vi "IMAQ FPGA Camera Link 8 Tap 10-Bit.vi"(6 "Ready for Output":bool=TRUE, 7 "Camera Link Enables":T3, 8 "Cancel Acquisition":bool, 9 "Acquire":bool=TRUE, 10 "Camera Link Data":T2, 11 "Acquisition Settings":T4) -> (0 "Output Valid":bool, 2 "Acquisition Status":T1, 3 "Vision Pixel Bus Out":T5={"Pixel Data"=[0, 0, 0, 0, 0, 0, 0, 0], "DV"=[FALSE, FALSE, FALSE, FALSE, FALSE, FALSE, FALSE, FALSE], "EOL"=FALSE, "EOI"=FALSE, "Data Type"=enum."U16 x 8"}, 5 "Acquisition Overflow":bool)   [LabVIEW 2017]
doc: "Acquires images from an 8 tap 10-bit (1X8-1Y) Camera Link Camera. On each pixel clock, 8 adjacent pixels arrive starting at the left of the image. Ensure that this VI is called from a Single Cycle Timed Loop that is running faster than the pixel clock of the camera.\n\nThe <B>Vision Pixel Bus Out</B> can be connected to Vision FPGA algorithms for processing."
uses:
  <vilib>/visionFPGA/Controls/IMAQ FPGA Pixel Bus u16x8.ctl
  <vilib>/visionFPGA/Basics/Camera Link Acquisition/Pixel Bus to Vision Pixel Bus/IMAQ FPGA Camera Link Pixel Bus to Vision Pixel Bus U16x8.vi
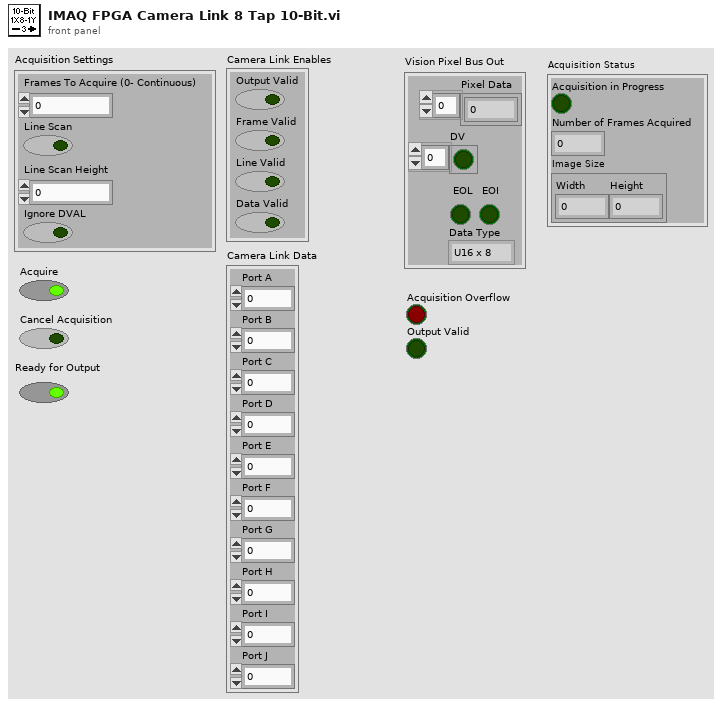
[diagram p1: front panel]
types:
  T1 = cluster{"Acquisition in Progress":bool, "Number of Frames Acquired":u32, "Image Size":cluster{"Width":u32, "Height":u32}}
  T2 = cluster{"Port A":u8, "Port B":u8, "Port C":u8, "Port D":u8, "Port E":u8, "Port F":u8, "Port G":u8, "Port H":u8, "Port I":u8, "Port J":u8}
  T3 = cluster{"Output Valid":bool, "Frame Valid":bool, "Line Valid":bool, "Data Valid":bool}
  T4 = cluster{"Frames To Acquire (0- Continuous)":u32, "Line Scan":bool, "Line Scan Height":u32, "Ignore DVAL":bool}
  T5 = typedef "IMAQ FPGA Pixel Bus u16x8.ctl" = cluster{"Pixel Data":u16[], "DV":bool[], "EOL":bool, "EOI":bool, "Data Type":enum16{"U16 x 8"}}
  T6 = cluster{"Acquisition in Progress":bool, "Num Frames Acquired":u32, "Height":u32, "Number of Cycles per Line":u32}
  T7 = cluster{"Acquisition in Progress":bool, "Num Frames Acquired":u32, cluster{u32, "Height":u32}}
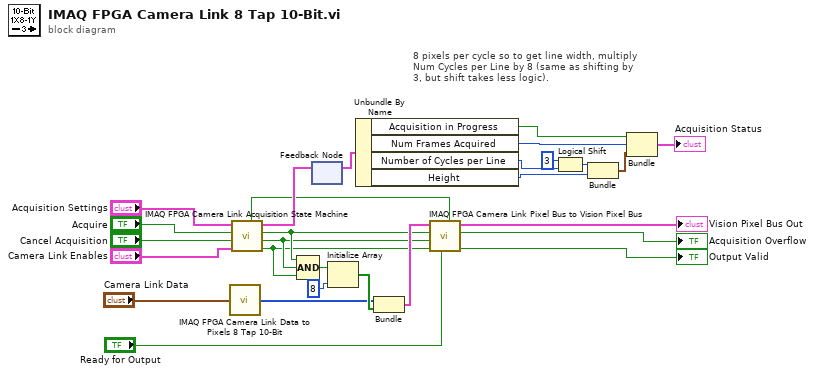
[diagram p0: block diagram]
diagram:
  # "8 pixels per cycle so to get line width, multiply Num Cycles per Line by 8 (same as shifting by 3, but shift takes less logic)."
  n1 = call <vilib>:"IMAQ FPGA Camera Link Data to Pixels 8 Tap 10-Bit.vi"("Camera Link Data"="Camera Link Data") -> ("Pixels"=w8:u16[])
  n2 = call <vilib>:"IMAQ FPGA Camera Link Acquisition State Machine.vi"("Enables"="Camera Link Enables", "Cancel Acq"="Cancel Acquisition", "Acquire"="Acquire", "Acquisition Settings"="Acquisition Settings") -> ("Output Valid"=w10:bool, "Frame Valid"=w11:bool, "Line Valid"=w12:bool, "Acquisition Status"=w27:T6, "Reset"=w5:bool)  [unwired: 3 in]
  n3 = Compound Arithmetic op=AND(w12, w11, w10) -> (w18:bool)
  n4 = feedback #1() -> (w26:T6)  [unwired: 1 in]
  n5 = feedback-in #1(w27) -> ()
  n6 = Initialize Array(w18, 8 ("dimension size")) -> (w17:bool[])
  n7 = Unbundle By Name(w26) -> ("Acquisition in Progress"=w3:bool, "Num Frames Acquired"=w4:u32, "Number of Cycles per Line"=w22:u32, "Height"=w28:u32)
  n8 = Bundle("Pixels"=w8, w17) -> (w16:cluster{"Pixels":u16[], bool[]})  [unwired: 1 in]
  n9 = call-poly <vilib>:"IMAQ FPGA Camera Link Pixel Bus to Vision Pixel Bus.vi"("Reset Overflow"=w5, "Ready for Output"="Ready for Output", "Input Valid"=w10, "Frame Valid In"=w11, "Line Valid In"=w12, "Pixel Bus x8 In"=w16) -> ("Output Valid"=→"Output Valid":bool, "Acquisition Overflow"=→"Acquisition Overflow":bool, "Vision Pixel Bus Out"=→"Vision Pixel Bus Out":T5)  [unwired: 3 in]
  n10 = Logical Shift(y=i16 3, x=w22) -> (x << y=w21:u32)
  n11 = Bundle(w21, "Height"=w28) -> (w2:cluster{u32, "Height":u32})  [unwired: 1 in]
  n12 = Bundle("Acquisition in Progress"=w3, "Num Frames Acquired"=w4, w2) -> (→"Acquisition Status":T7)  [unwired: 1 in]
